vi "HandleElevatedPass.vi"(7 "InitState":T1, 8 "error in (no error)":errorcluster, 11 "Toggle?":bool) -> (0 "error out":errorcluster, 3 "PassState":T1)   [LabVIEW 2013]
uses:
  PassState.ctl
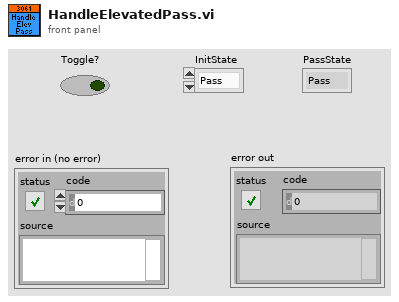
[diagram p1: front panel]
types:
  T1 = typedef "PassState.ctl" = enum16{"Pass", "Stop"}
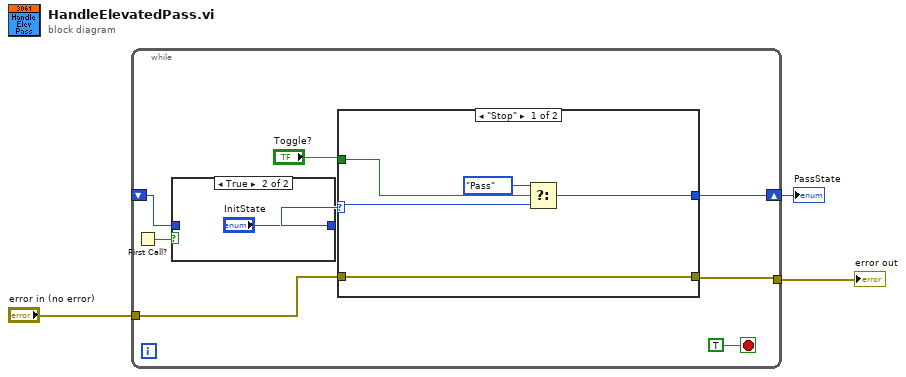
[diagram p0: block diagram]
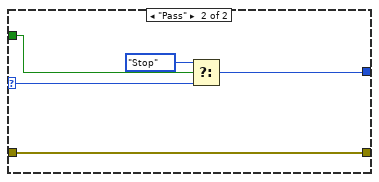
[diagram p3: hidden frame]
diagram:
  n1 = while {
    tunnel: "error in (no error)" -> [w9]
    tunnel: [w8] -> w2
    shift-right: [w6] -> w1
    shift-left: _ -> [w5]
    stop <- TRUE stop-if-true
    n2 = First Call?() -> (First Call?: T/F=w10:bool)
    n3 = case shown="True" w10 {
      tunnel: [w12 "InitState"] -> w7
      tunnel: w5 -> [w12 _]
      frame False {
      }
      frame True {
      }
    }
    n4 = case shown="\"Stop\"" w7 {
      selector: w7 -> [w17 w23]
      tunnel: w9 -> [w18 w21]
      tunnel: [w18 w21] -> w8
      tunnel: [w16 w22] -> w6
      tunnel: "Toggle?" -> [w15 w20]
      frame "Stop" {
        n5 = Select(t=PassState."Pass", s=w15, f=w17) -> (s? t:f=w16:T1)
      }
      frame "Pass" {
        n6 = Select(t=PassState."Stop", s=w20, f=w23) -> (s? t:f=w22:T1)
      }
    }
  }
  "error out" <- w2
  "PassState" <- w1
